vi "Write PFX Certificate.vi"(8 "error in (no error)":errorcluster, 10 "PFX Certificate":path, 11 "dotNET SSL Socket in":refnum<class "dotNET SSL Server.lvclass">) -> (0 "error out":errorcluster, 3 "dotNET SSL Socket out":refnum<class "dotNET SSL Server.lvclass">)   [LabVIEW 2013, in "dotNET SSL Socket.lvlib" / "dotNET SSL Server.lvclass"]
uses:
  dotNET SSL Server/dotNET SSL Server.lvclass
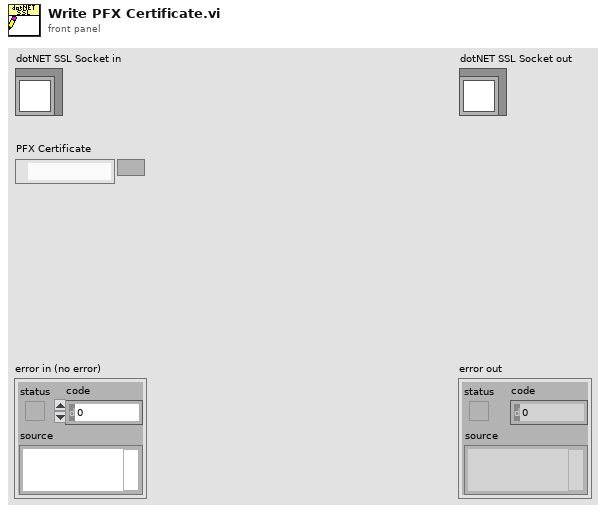
[diagram p1: front panel]
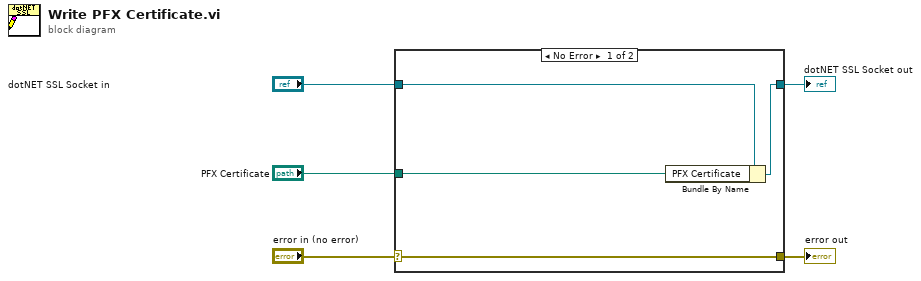
[diagram p0: block diagram]
diagram:
  n1 = case shown="No Error" "error in (no error)" {
    selector: "error in (no error)" -> [w9 w10]
    tunnel: [w9 w10] -> w4
    tunnel: [w7 w11] -> w2
    tunnel: "dotNET SSL Socket in" -> [w8 w11]
    tunnel: "PFX Certificate" -> [w6 _]
    frame No Error {
      n2 = Bundle By Name(cluster=w8, "PFX Certificate"=w6) -> (w7:refnum<class "dotNET SSL Server.lvclass">)
    }
    frame Error {
    }
  }
  "error out" <- w4
  "dotNET SSL Socket out" <- w2
